vi "Bodies_GetGravityVecInXYZ0.vi"(6 "Input is Weight (F)":bool, 8 "error in (no error)":errorcluster, 9 "Mass(kg)":dbl, 11 "Bodies in":refnum<class "Bodies.lvclass">) -> (0 "error out":errorcluster, 1 "GravityVector":dbl[](array[numeric]), 3 "Bodies out":refnum<class "Bodies.lvclass">)   [LabVIEW 2015, in "Bodies.lvclass"]
uses:
  Bodies.lvclass
  Bodies.lvclass/Bodies.ctl
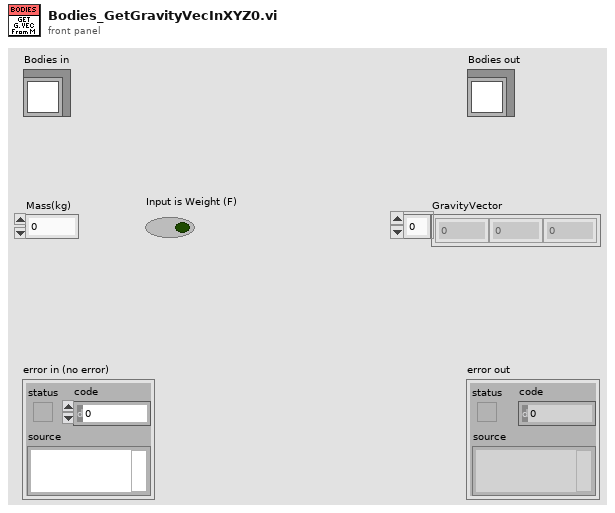
[diagram p1: front panel]
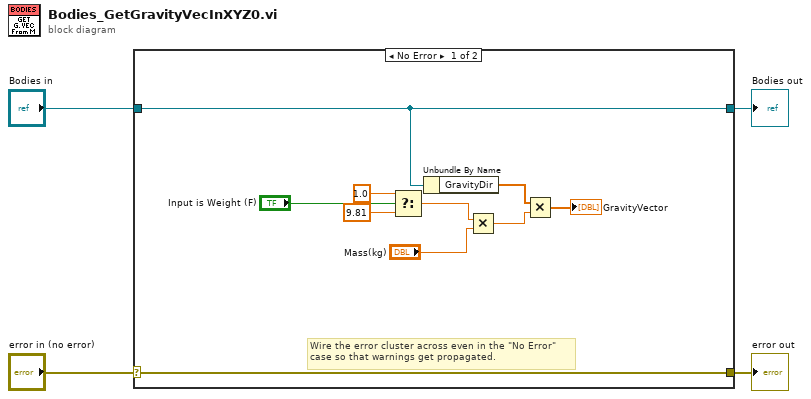
[diagram p0: block diagram]
diagram:
  n1 = case shown="No Error" "error in (no error)" {
    selector: "error in (no error)" -> [w14 w16]
    tunnel: [w14 w16] -> w3
    tunnel: [w8 w15] -> w1
    tunnel: "Bodies in" -> [w8 w15]
    frame No Error {
      # "Wire the error cluster across even in the \"No Error\"\ncase so that warnings get propagated."
      n2 = Select(t=1.0, s="Input is Weight (F)", f=9.81) -> (s? t:f=w12:dbl)
      n3 = Unbundle By Name(w8) -> ("GravityDir"=w7:dbl[])
      n4 = Multiply(x=w12, y="Mass(kg)") -> (x*y=w6:dbl)
      n5 = Multiply(x=w7, y=w6) -> (x*y=→"GravityVector":dbl[])
    }
    frame Error {
    }
  }
  "error out" <- w3
  "Bodies out" <- w1
